vi "EXO2全局变量.vi"() -> ()   [LabVIEW 2016, in "EXO2.lvlib"]
uses:
  EXO2.lvlib
panel:
  out "EXO message Array":T1(array[cluster])
  out "EXO message":T2
  in  "EXO2baud rate (9600)":u32=9600
  in  "EXO2串口":refnum<visa-resource-name>="COM9"
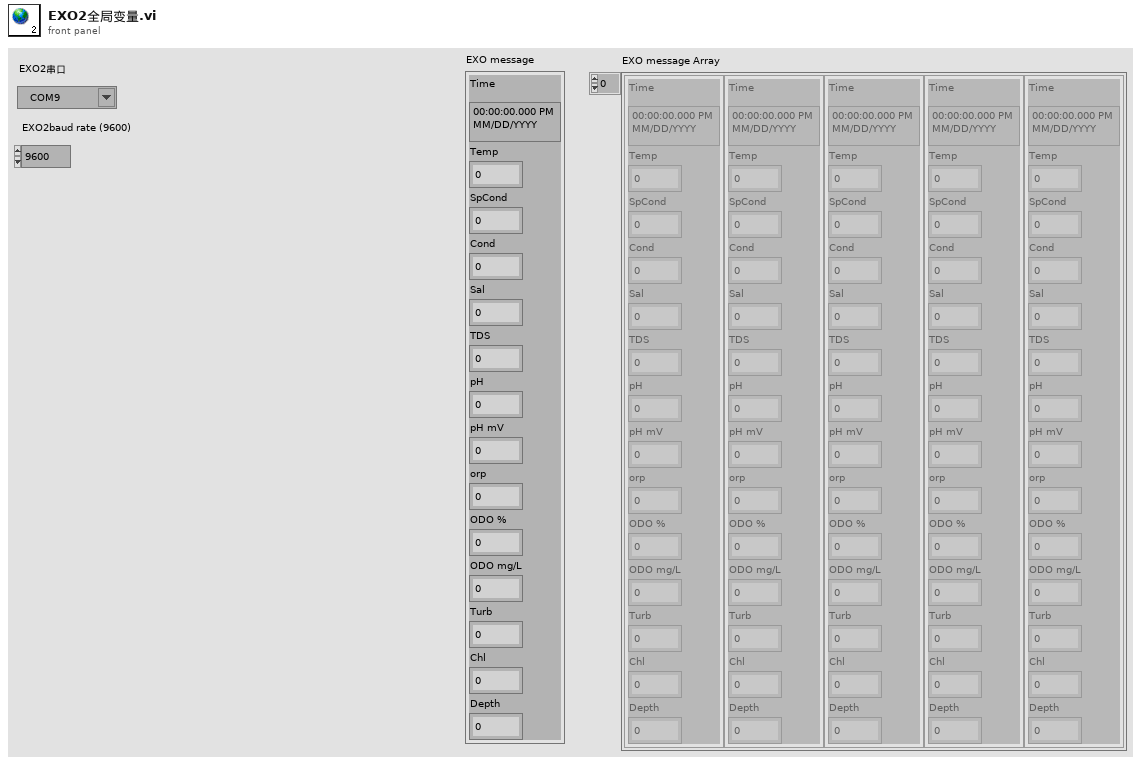
[diagram p1: front panel]
types:
  T1 = cluster{"Time":timestamp, "Temp":dbl, "SpCond":dbl, "Cond":dbl, "Sal":dbl, "TDS":dbl, "pH":dbl, "pH mV":dbl, "orp":dbl, "ODO %":dbl, "ODO mg/L":dbl, "Turb":dbl, "Chl":dbl, "Depth":dbl}[]
  T2 = cluster{"Time":timestamp, "Temp":dbl, "SpCond":dbl, "Cond":dbl, "Sal":dbl, "TDS":dbl, "pH":dbl, "pH mV":dbl, "orp":dbl, "ODO %":dbl, "ODO mg/L":dbl, "Turb":dbl, "Chl":dbl, "Depth":dbl}
diagram:
